vi "GetChildByName.vi"(8 "error in (no error)":errorcluster, 10 "BrowerComponentID(\"\")":string, 11 "reference in":refnum<class "BrowerComposite.lvclass">) -> (0 "error out":errorcluster, 2 "BrowerComponent":refnum<class "BrowerComponent.lvclass">, 3 "reference out":refnum<class "BrowerComposite.lvclass">)   [LabVIEW 2015, in "BrowerComposite.lvclass"]
uses:
  BrowerComposite.lvclass
  BrowerComponent/BrowerComponent.lvclass
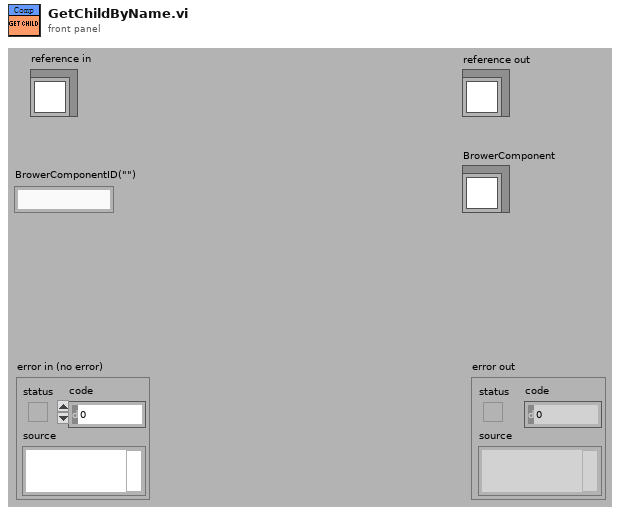
[diagram p1: front panel]
types:
  T1 = typedef "BrowerComposite.lvclass/ObjectAttributes.ctl" = cluster{"BrowerComponents":refnum<class "BrowerComponent.lvclass">[], "BrowerComponentIDs":string[], "Iterator":refnum<class "Iterator.lvclass">}
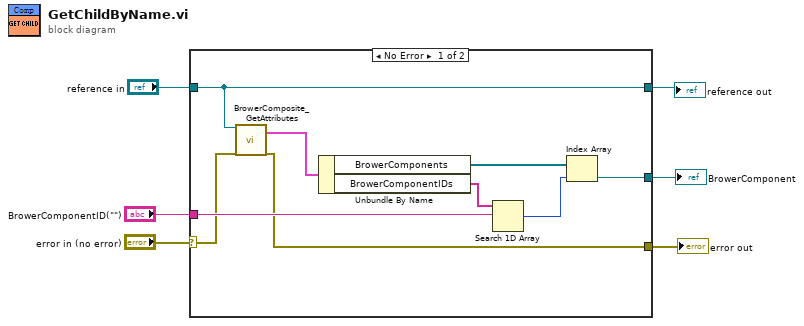
[diagram p0: block diagram]
diagram:
  n1 = case shown="No Error" "error in (no error)" {
    selector: "error in (no error)" -> [w8 w17]
    tunnel: "BrowerComponentID(\"\")" -> [w13 _]
    tunnel: [w10 _] -> w5
    tunnel: "reference in" -> [w7 w16]
    tunnel: [w9 w17] -> w3
    tunnel: [w7 w16] -> w1
    frame No Error {
      n2 = call "BrowerComposite_GetAttributes.vi"("reference in"=w7, "error in (no error)"=w8) -> ("Data"=w15:T1, "error out"=w9:errorcluster)  [unwired: 14 in, 2 out]
      n3 = Unbundle By Name(w15) -> ("BrowerComponents"=w12:refnum<class "BrowerComponent.lvclass">[], "BrowerComponentIDs"=w14:string[])
      n4 = Search 1D Array(1D array=w14, element=w13) -> (index of element=w11:i32)  [unwired: 1 in]
      n5 = Index Array(array=w12, index=w11) -> (element=w10:refnum<class "BrowerComponent.lvclass">)
    }
    frame Error {
    }
  }
  "error out" <- w3
  "reference out" <- w1
  "BrowerComponent" <- w5
